vi "Asynchronous Logger.vi"(8 "error in (no error)":errorcluster, 9 "Test Modes":string[](array[string]), 10 "Limits File Path":path, 11 "QMH Queue":refnum<queue>) -> (0 "error out":errorcluster)   [LabVIEW 2018, in "Test Number and Bin Generator.lvlib" / "Test Number and Bin Generator.lvclass"]
uses:
  Test Number and Bin Generator.lvclass
  Typedefs/Evaluation QMH.ctl
  Plugins/TestStand API Tools (TSAT).lvlibp/Evaluation Actions/Includes/Controls/TSAT Eval SI Unit Scaling.ctl
  Plugins/TestStand API Tools (TSAT).lvlibp/Evaluation Actions/Includes/Controls/TSAT Evaluation Type.ctl
  Plugins/TestStand API Tools (TSAT).lvlibp/Evaluation Actions/TSAT Evaluation Actions.lvlib
panel:
  out "Numeric":i32
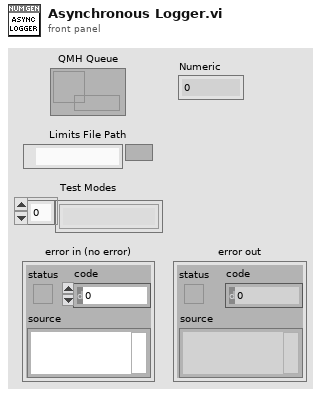
[diagram p1: front panel]
types:
  T1 = typedef "Test Number and Bin Generator.lvlib/Test Number and Bin Generator.lvclass/Evaluation QMH.ctl" = cluster{"Command":string, "Evaluations":cluster{"Test Name":string, "Pin":string, "Units":string, "SI Scaling":T2, "Test Number":i32, "Published Data Id":string, "Low Limit":dbl, "High Limit":dbl, "Export Data Location":string, "Software Bin":i64, "Evaluation Type":T3, "Test Data Source":string}[]}
  T2 = typedef "TestStand API Tools (TSAT).lvlibp/TSAT Evaluation Actions.lvlib/TSAT Eval SI Unit Scaling.ctl" = i16
  T3 = typedef "TestStand API Tools (TSAT).lvlibp/TSAT Evaluation Actions.lvlib/TSAT Evaluation Type.ctl" = enum16{"Numeric Limit", "Pass/Fail", "None"}
  T4 = cluster{"Test Name":string, "Pin":string, "Units":string, "SI Scaling":T2, "Test Number":i32, "Published Data Id":string, "Low Limit":dbl, "High Limit":dbl, "Export Data Location":string, "Software Bin":i64, "Evaluation Type":T3, "Test Data Source":string}[]
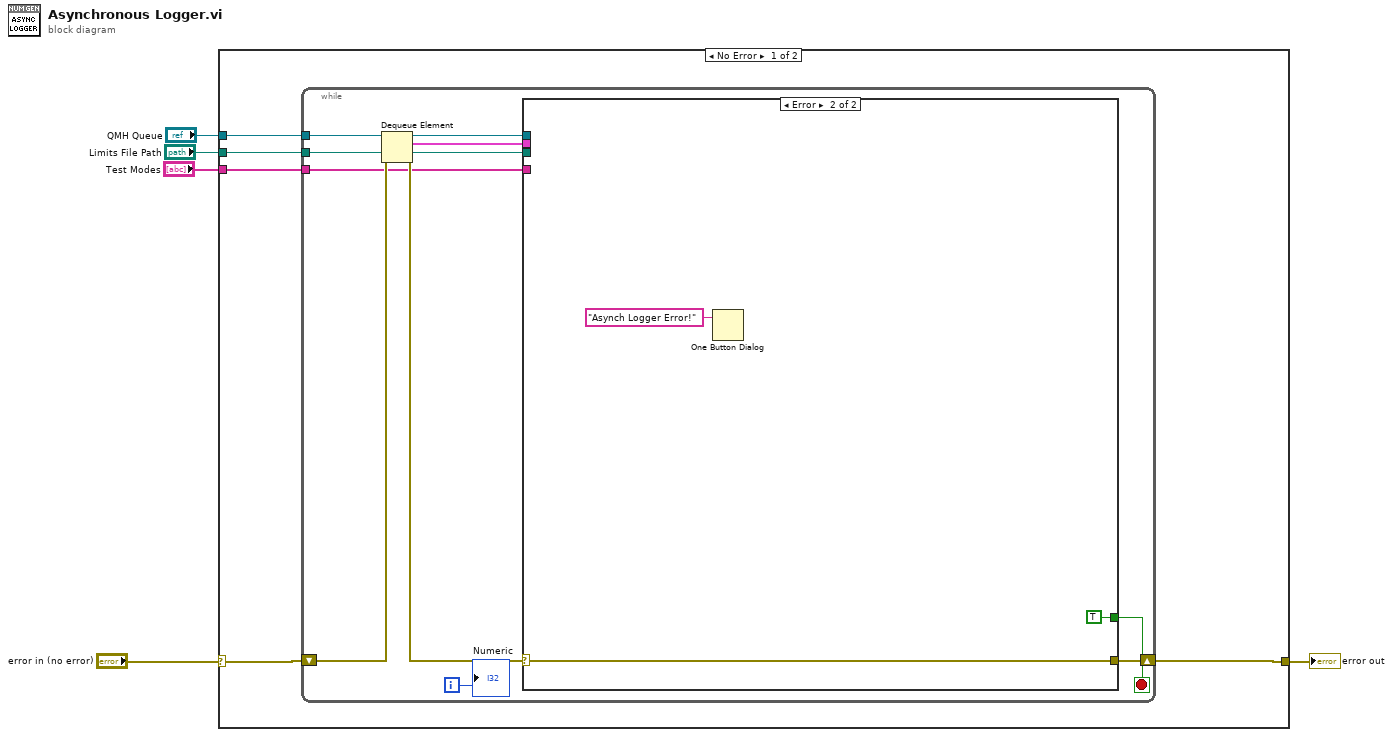
[diagram p0: block diagram]
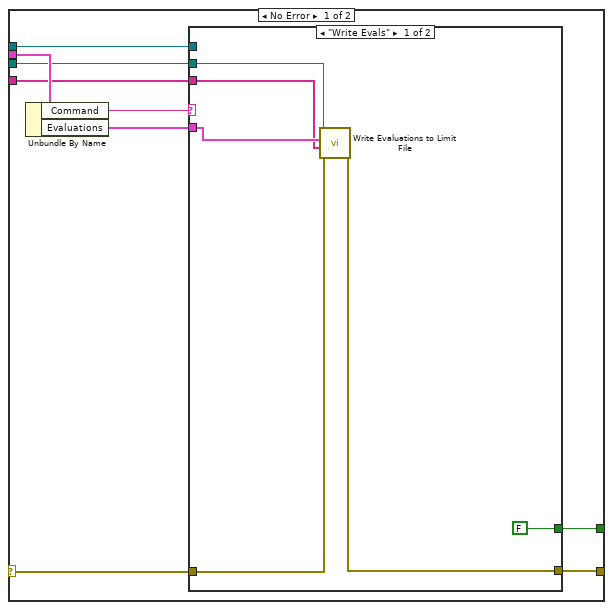
[diagram p2: hidden frame]
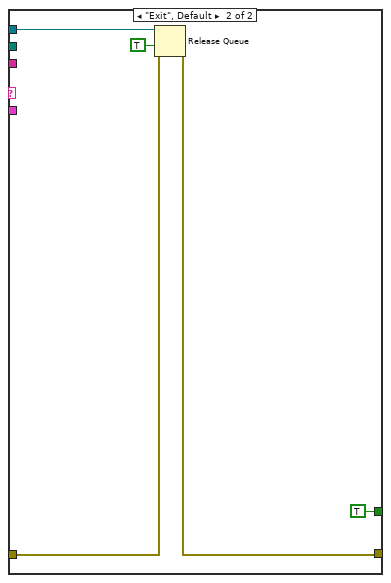
[diagram p3: hidden frame]
diagram:
  n1 = case shown="No Error" "error in (no error)" {
    selector: "error in (no error)" -> [w10 w44]
    tunnel: [w9 w44] -> w4
    tunnel: "QMH Queue" -> [w8 _]
    tunnel: "Limits File Path" -> [w7 _]
    tunnel: "Test Modes" -> [w6 _]
    frame No Error {
      n2 = while {
        shift-right: [w17] -> w9
        shift-left: w10 -> [w19]
        tunnel: w7 -> [w14]
        tunnel: w6 -> [w13]
        tunnel: w8 -> [w20]
        i -> [w11]
        stop <- w15 stop-if-true
        n3 = Dequeue Element(queue=w20, error in (no error)=w19) -> (queue out=w12:refnum<queue>, element=w16:T1, error out=w18:errorcluster)  [unwired: 1 in, 1 out]
        n4 = case shown="Error" w18 {
          selector: w18 -> [w26 w43]
          tunnel: [w25 w43] -> w17
          tunnel: w16 -> [w29 _]
          tunnel: [w24 TRUE] -> w15
          tunnel: w14 -> [w23 _]
          tunnel: w13 -> [w22 _]
          tunnel: w12 -> [w21 _]
          frame No Error {
            n5 = Unbundle By Name(w29) -> ("Command"=w28:string, "Evaluations"=w27:T4)
            n6 = case shown="\"Write Evals\"" w28 {
              tunnel: w27 -> [w35 _]
              tunnel: w26 -> [w34 w40]
              tunnel: [w33 w39] -> w25
              tunnel: [FALSE TRUE] -> w24
              tunnel: w23 -> [w31 _]
              tunnel: w22 -> [w30 _]
              tunnel: w21 -> [_ w37]
              frame "Write Evals" {
                n7 = call "Write Evaluations to Limit File.vi"("error in (no error)"=w34, "Test Modes"=w30, "Evaluations In"=w35, "Limits File Path"=w31) -> ("error out"=w33:errorcluster)  [unwired: 7 in]
              }
              frame "Exit", Default {
                n8 = Release Queue(queue=w37, force destroy? (F)=TRUE, error in (no error)=w40) -> (error out=w39:errorcluster)  [unwired: 2 out]
              }
            }
          }
          frame Error {
            n9 = One Button Dialog(message="Asynch Logger Error!") -> ()  [unwired: 1 in, 1 out]
          }
        }
        "Numeric" <- w11
      }
    }
    frame Error {
    }
  }
  "error out" <- w4
